vi "FPGA Voltage Input Write.vi"(8 "error in (no error)":errorcluster, 11 "RT data in":T1) -> (0 "error out":errorcluster, 3 "RT data out":T1)   [LabVIEW 2011, in "Engine Sim RT.lvlib"]
uses:
  Engine Sim RT.lvlib
  TypeDefs/RT Data Cluster.ctl
  Shared/Channel Descriptors.ctl
  Shared/FPGA Write Descriptor.ctl
  Shared/InputChannelTypes.ctl
  <vilib>/rvi/DataTransferAndStorage/Container/Common/niFpgaDataTypeControl.ctl
  Shared/FPGA Read Descriptor.ctl
  Shared/OutputChannelTypes.ctl
  Shared/Status Chan Descriptor.ctl
  Shared/DataReplayVoltageConfig.ctl
  <userlib>/_FPGA Interface Advanced Tools/FPGA Interface Wrapper/NiFPGA Write - U32.vi
  <userlib>/_FPGA Interface Advanced Tools/FPGA Interface Wrapper/NiFPGA Write - I32.vi
  <vilib>/Utility/error.llb/Error Cluster From Error Code.vi
  <userlib>/_FPGA Interface Advanced Tools/FPGA Interface Wrapper/FPGA Interface Wrapper.lvlib
  Engine Simulation Shared.lvlib
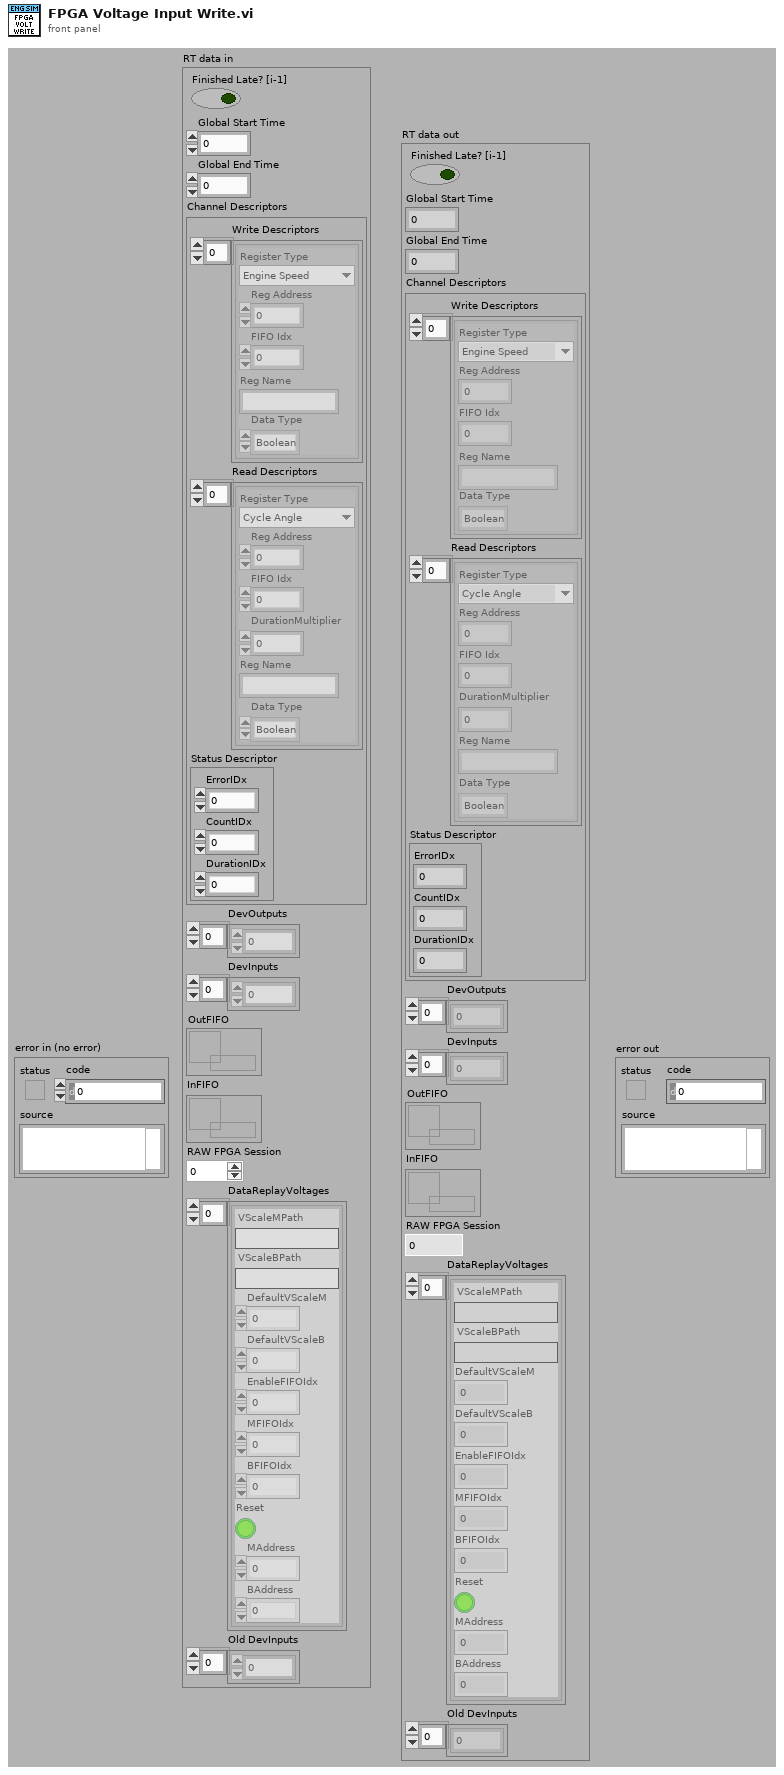
[diagram p1: front panel]
types:
  T1 = typedef "Engine Sim RT.lvlib/RT Data Cluster.ctl" = cluster{"Finished Late? [i-1]":bool, "Global Start Time":i64, "Global End Time":i64, "Channel Descriptors":T2, "DevOutputs":dbl[], "DevInputs":dbl[], "OutFIFO":refnum<k33>, "InFIFO":refnum<k33>, "RAW FPGA Session":u32, "DataReplayVoltages":T9[], "Old DevInputs":dbl[]}
  T2 = typedef "Engine Simulation Shared.lvlib/Channel Descriptors.ctl" = cluster{"Write Descriptors":T3[], "Read Descriptors":T6[], "Status Descriptor":T8}
  T3 = typedef "Engine Simulation Shared.lvlib/FPGA Write Descriptor.ctl" = cluster{"Register Type":T4, "Reg Address":u32, "FIFO Idx":i32, "Reg Name":string, "Data Type":T5}
  T4 = typedef "Engine Simulation Shared.lvlib/InputChannelTypes.ctl" = enum16{"Engine Speed", "Offset"}
  T5 = typedef "niFpgaDataTypeControl.ctl" = enum32{"Boolean", "I8", "I16", "I32", "I64", "U8", "U16", "U32", "U64", "FXP", "CustomControl"}
  T6 = typedef "Engine Simulation Shared.lvlib/FPGA Read Descriptor.ctl" = cluster{"Register Type":T7, "Reg Address":u32, "FIFO Idx":i32, "DurationMultiplier":dbl, "Reg Name":string, "Data Type":T5}
  T7 = typedef "Engine Simulation Shared.lvlib/OutputChannelTypes.ctl" = enum16{"Cycle Angle", "Crank Angle", "Time Duration", "Angle Duration", "Start Angle", "End Angle"}
  T8 = typedef "Engine Simulation Shared.lvlib/Status Chan Descriptor.ctl" = cluster{"ErrorIDx":i32, "CountIDx":i32, "DurationIDx":i32}
  T9 = typedef "Engine Simulation Shared.lvlib/DataReplayVoltageConfig.ctl" = cluster{"VScaleMPath":string, "VScaleBPath":string, "DefaultVScaleM":u32, "DefaultVScaleB":i32, "EnableFIFOIdx":i32, "MFIFOIdx":i32, "BFIFOIdx":i32, "Reset":bool, "MAddress":u32, "BAddress":u32}
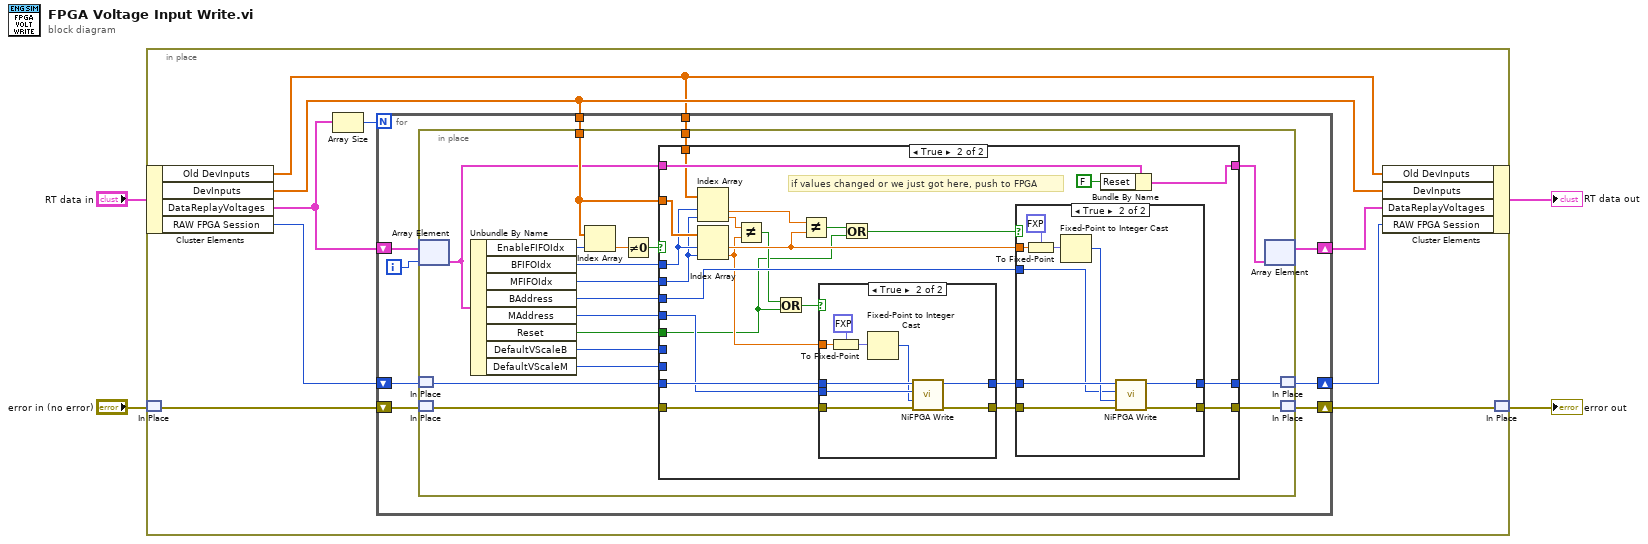
[diagram p0: block diagram]
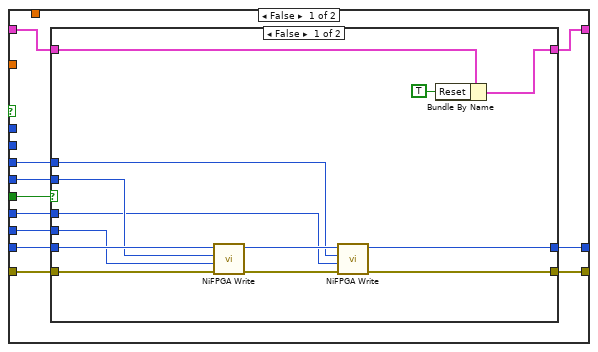
[diagram p2: hidden frame]
diagram:
  n1 = in-place {
    n2 = in-place-cluster #1("RT data in") -> ("Old DevInputs"=w5:dbl[], "DevInputs"=w6:dbl[], "DataReplayVoltages"=w10:T9[], "RAW FPGA Session"=w9:u32)
    n3 = in-place-match #2("error in (no error)") -> (w12:errorcluster)
    n4 = Array Size(array=w10) -> (size(s)=w13:i32)
    n5 = for {
      N: w13 -> [_]
      tunnel: w6 -> [w22]
      shift-right: [w19] -> w7
      shift-left: w10 -> [w21]
      shift-right: [w17] -> w8
      shift-left: w9 -> [w16]
      shift-right: [w18] -> w11
      shift-left: w12 -> [w15]
      tunnel: w5 -> [w14]
      i -> [w20]
      n6 = in-place {
        in-place-border: w22 -> [w32]
        in-place-border: w14 -> [w23]
        n7 = in-place-array #3(w21, w20) -> (w29:T9)
        n8 = in-place-match #4(w16) -> (w25:u32)
        n9 = in-place-match #5(w15) -> (w24:errorcluster)
        n10 = Unbundle By Name(w29) -> ("EnableFIFOIdx"=w40:i32, "BFIFOIdx"=w37:i32, "MFIFOIdx"=w36:i32, "BAddress"=w34:u32, "MAddress"=w35:u32, "Reset"=w33:bool, "DefaultVScaleB"=w30:i32, "DefaultVScaleM"=w31:u32)
        n11 = Index Array(array=w32, index=w40) -> (element=w39:dbl)
        n12 = Not Equal To 0?(x=w39) -> (x != 0?=w38:bool)
        n13 = case shown="True" w38 {
          tunnel: w24 -> [w49 w91]
          tunnel: [w50 w89] -> w27
          tunnel: w25 -> [w48 w88]
          tunnel: [w47 w86] -> w26
          tunnel: w32 -> [_ w85]
          tunnel: w37 -> [_ w78]
          tunnel: w36 -> [_ w77]
          tunnel: w35 -> [w43 w84]
          tunnel: w34 -> [w41 w83]
          tunnel: w33 -> [w51 w68]
          tunnel: w29 -> [w46 w82]
          tunnel: [w45 w81] -> w28
          tunnel: w31 -> [w44 _]
          tunnel: w30 -> [w42 _]
          tunnel: w23 -> [_ w79]
          frame False {
            n14 = case shown="False" w51 {
              tunnel: [w57 w67] -> w50
              tunnel: w49 -> [w58 w67]
              tunnel: w48 -> [w59 w66]
              tunnel: [w56 w66] -> w47
              tunnel: w46 -> [w64 w65]
              tunnel: [w62 w65] -> w45
              tunnel: w44 -> [w55 _]
              tunnel: w43 -> [w54 _]
              tunnel: w42 -> [w53 _]
              tunnel: w41 -> [w52 _]
              frame False {
                n15 = call-poly <userlib>:"NiFPGA Write.vi"("error in (no error)"=w58, "Value"=w55, "Control"=w54, "Session"=w59) -> ("error out"=w61:errorcluster, "Session Out"=w60:u32)  [unwired: 6 in]
                n16 = call-poly <userlib>:"NiFPGA Write.vi"("error in (no error)"=w61, "Value"=w53, "Control"=w52, "Session"=w60) -> ("error out"=w57:errorcluster, "Session Out"=w56:u32)  [unwired: 6 in]
                n17 = Bundle By Name(cluster=w64, "Reset"=TRUE) -> (w62:T9)
              }
              frame True {
              }
            }
          }
          frame True {
            # "if values changed or we just got here, push to FPGA"
            n18 = Index Array(array=w79, index #1=w78, index #2=w77) -> (element #1=w76:dbl, element #2=w74:dbl)
            n19 = Index Array(array=w85, index #1=w78, index #2=w77) -> (element #1=w75:dbl, element #2=w73:dbl)
            n20 = Not Equal?(x=w74, y=w73) -> (x != y?=w72:bool)
            n21 = Or(x=w72, y=w68) -> (x .or. y?=w71:bool)
            n22 = Not Equal?(x=w76, y=w75) -> (x != y?=w69:bool)
            n23 = case shown="True" w71 {
              tunnel: w91 -> [w92 w102]
              tunnel: [w92 w101] -> w90
              tunnel: w88 -> [w93 w100]
              tunnel: [w93 w99] -> w87
              tunnel: w84 -> [_ w98]
              tunnel: w73 -> [_ w97]
              frame False {
              }
              frame True {
                n24 = To Fixed-Point(fixed-point type=fxp<+,18,12> 0.0, number=w97) -> (fixed-point=w96:fxp<+,18,12>)
                n25 = Fixed-Point to Integer Cast(1:w96) -> (0:w95:u32)
                n26 = call-poly <userlib>:"NiFPGA Write.vi"("error in (no error)"=w102, "Value"=w95, "Control"=w98, "Session"=w100) -> ("error out"=w101:errorcluster, "Session Out"=w99:u32)  [unwired: 6 in]
              }
            }
            n27 = Or(x=w69, y=w68) -> (x .or. y?=w70:bool)
            n28 = case shown="True" w70 {
              tunnel: w90 -> [w104 w113]
              tunnel: [w104 w112] -> w89
              tunnel: w87 -> [w103 w111]
              tunnel: [w103 w110] -> w86
              tunnel: w75 -> [_ w108]
              tunnel: w83 -> [_ w105]
              frame False {
              }
              frame True {
                n29 = To Fixed-Point(fixed-point type=fxp<+/-,18,3> 0.0, number=w108) -> (fixed-point=w107:fxp<+/-,18,3>)
                n30 = Fixed-Point to Integer Cast(1:w107) -> (0:w106:i32)
                n31 = call-poly <userlib>:"NiFPGA Write.vi"("error in (no error)"=w113, "Value"=w106, "Control"=w105, "Session"=w111) -> ("error out"=w112:errorcluster, "Session Out"=w110:u32)  [unwired: 6 in]
              }
            }
            n32 = Bundle By Name(cluster=w82, "Reset"=FALSE) -> (w81:T9)
          }
        }
        n33 = in-place-array #3(w28) -> (w19:T9[])  [unwired: 1 out]
        n34 = in-place-match #4(w26) -> (w17:u32)
        n35 = in-place-match #5(w27) -> (w18:errorcluster)
      }
    }
    n36 = in-place-cluster #1("Old DevInputs"=w5, "DevInputs"=w6, "DataReplayVoltages"=w7, "RAW FPGA Session"=w8) -> (→"RT data out":T1)
    n37 = in-place-match #2(w11) -> (→"error out":errorcluster)
  }
